vi "ViHandler.Exit.vi"(8 "error in (no error)":errorcluster, 11 "ViHandler in":refnum<class "ViHandler.lvclass">) -> (0 "error out":errorcluster, 3 "ViHandler out":refnum<class "ViHandler.lvclass">)   [LabVIEW 2016, in "ViHandler.lvclass"]
uses:
  ViHandler.lvclass
  ViHandler.ViInfo.ctl
  ViHandler.lvclass/ViHandler.ctl
panel:
  out "Array":T1[](array[typedef])
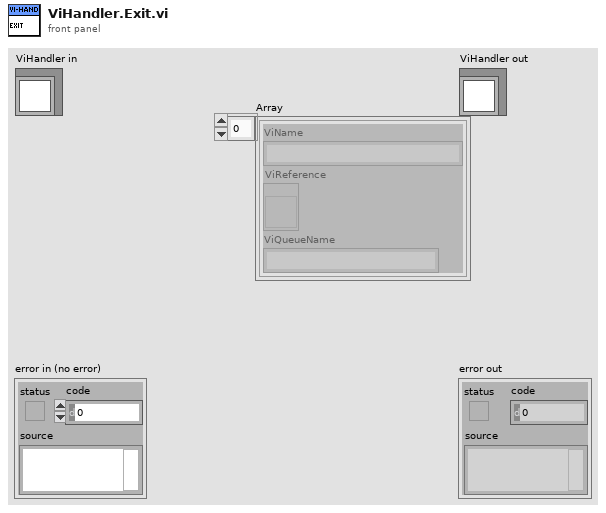
[diagram p1: front panel]
types:
  T1 = typedef "ViHandler.lvclass/ViHandler.ViInfo.ctl" = cluster{"ViName":string, "ViReference":refnum<vi>, "ViQueueName":string}
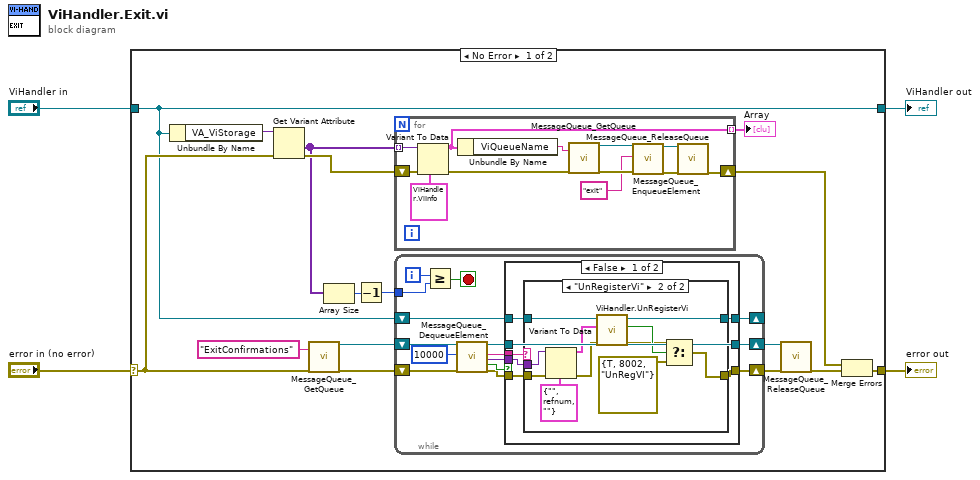
[diagram p0: block diagram]
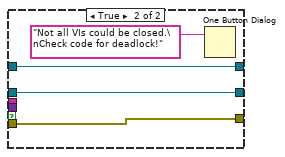
[diagram p3: hidden frame]
diagram:
  n1 = case shown="No Error" "error in (no error)" {
    selector: "error in (no error)" -> [w17 w73]
    tunnel: [w11 w73] -> w3
    tunnel: [w6 w72] -> w1
    tunnel: "ViHandler in" -> [w6 w72]
    frame No Error {
      n2 = Unbundle By Name(w6) -> ("VA_ViStorage"=w20:variant)
      n3 = Get Variant Attribute(Variant=w20, error in=w17) -> (values=w14:variant[], error out=w19:errorcluster)  [unwired: 2 in, 2 out]
      n4 = call "MessageQueue_GetQueue.vi"("Name"="ExitConfirmations", "ErrorIn"=w17) -> ("QueueOut"=w15:refnum<queue>, "ErrorOut"=w16:errorcluster)  [unwired: 15 in, 1 out]
      n5 = Array Size(array=w14) -> (size(s)=w13:i32)
      n6 = Decrement(x=w13) -> (x-1=w12:i32)
      n7 = for {
        tunnel: w14 -> [w71] mode=indexing
        shift-right: [w65] -> w10
        shift-left: w19 -> [w70]
        tunnel: [w60] -> w5 mode=indexing
        n8 = Variant To Data(error in=w70, type=T1 {"ViName"="MultiChamberInterfaceUI.vi", "ViReference"=refnum, "ViQueueName"="MultiChamberInterfaceUI"} ("ViInfo"), Variant=w71) -> (data=w60:T1, error out=w66:errorcluster)
        n9 = Unbundle By Name(w60) -> ("ViQueueName"=w64:string)
        n10 = call "MessageQueue_GetQueue.vi"("Name"=w64, "ErrorIn"=w66) -> ("QueueOut"=w63:refnum<queue>, "ErrorOut"=w67:errorcluster)  [unwired: 15 in, 1 out]
        n11 = call "MessageQueue_EnqueueElement.vi"("QueueIn"=w63, "Message"="exit", "ErrorIn"=w67) -> ("QueueOut"=w62:refnum<queue>, "ErrorOut"=w68:errorcluster)  [unwired: 15 in]
        n12 = call "MessageQueue_ReleaseQueue.vi"("QueueIn"=w62, "ErrorIn"=w68) -> ("ErrorOut"=w65:errorcluster)  [unwired: 15 in, 2 out]
      }
      "Array" <- w5
      n13 = while {
        shift-right: [w26] -> w8
        shift-left: w16 -> [w31]
        shift-right: [w25] -> w9
        shift-left: w15 -> [w32]
        tunnel: w12 -> [w35]
        shift-right: [w21] -> _
        shift-left: w6 -> [w22]
        i -> [w34]
        stop <- w33 stop-if-true
        n14 = Greater Or Equal?(x=w34, y=w35) -> (x >= y?=w33:bool)
        n15 = call "MessageQueue_DequeueElement.vi"("QueueIn"=w32, "Timeout"=10000, "ErrorIn"=w31) -> ("QueueOut"=w27:refnum<queue>, "Message"=w24:string, "Data"=w23:variant, "Timeout"=w29:bool, "ErrorOut"=w28:errorcluster)  [unwired: 12 in]
        n16 = case shown="False" w29 {
          tunnel: w28 -> [w39 w59]
          tunnel: w27 -> [w42 w58]
          tunnel: [w38 w59] -> w26
          tunnel: [w42 w58] -> w25
          tunnel: w24 -> [w41 _]
          tunnel: w23 -> [w40 _]
          tunnel: w22 -> [w37 w56]
          tunnel: [w36 w56] -> w21
          frame False {
            n17 = case shown="\"UnRegisterVi\"" w41 {
              tunnel: w40 -> [_ w54]
              tunnel: w39 -> [w44 w55]
              tunnel: [w44 w45] -> w38
              tunnel: w37 -> [w43 w52]
              tunnel: [w43 w51] -> w36
              frame Default {
              }
              frame "UnRegisterVi" {
                n18 = Variant To Data(error in=w55, type=T1 {"ViName"="", "ViReference"=refnum, "ViQueueName"=""} ("ViInfo"), Variant=w54) -> (data=w50:T1, error out=w49:errorcluster)
                n19 = call "ViHandler.UnRegisterVi.vi"("error in (no error)"=w49, "ViInfo"=w50, "ViHandler in"=w52) -> ("error out"=w47:errorcluster, "UnregisterSuccessful?"=w48:bool, "ViHandler out"=w51:refnum<class "ViHandler.lvclass">)  [unwired: 6 in]
                n20 = Select(t=w47, s=w48, f=errorcluster {"status"=TRUE, "code"=8002, "source"="UnRegVI"}) -> (s? t:f=w45:errorcluster)
              }
            }
          }
          frame True {
            n21 = One Button Dialog(message="Not all VIs could be closed.\nCheck code for deadlock!") -> ()  [unwired: 1 in, 1 out]
          }
        }
      }
      n22 = call "MessageQueue_ReleaseQueue.vi"("QueueIn"=w9, "ErrorIn"=w8) -> ("ErrorOut"=w7:errorcluster)  [unwired: 15 in, 2 out]
      n23 = Merge Errors(w10, w7) -> (w11:errorcluster)
    }
    frame Error {
    }
  }
  "error out" <- w3
  "ViHandler out" <- w1
